vi "ATSh_WaitNextAsyncBufferComplete.vi"(8 "uTimeout_ms":u32, 9 "uBytesPerBuffer":u32, 10 "pBuffer_In":u16[](array[numeric]), 11 "Handle":u32) -> (0 "Return Code":u32, 2 "pBuffer_Out":u16[](array[numeric]), 3 "Handle_Out":u32)   [LabVIEW 2015]
doc: "_____AlazarTech, Scope_____\n\nWait for an asynchronous transfer from on-board to host memory to complete."
uses:
  ATSApi.dll
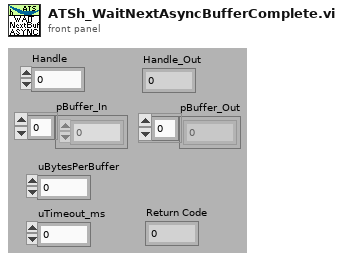
[diagram p1: front panel]
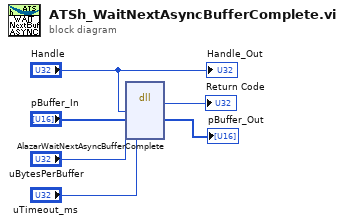
[diagram p0: block diagram]
diagram:
  n1 = dll-call lib="C:/IntensityOCT/trunk/ATSApi.dll" fn="AlazarWaitNextAsyncBufferComplete"("Handle"="Handle", "pBuffer"="pBuffer_In", "uBytesPerBuffer"="uBytesPerBuffer", "uTimeout_ms"="uTimeout_ms") -> (→"Return Code":u32, "pBuffer"=→"pBuffer_Out":u16[])  [unwired: 6 in, 2 out]
  "Handle_Out" <- "Handle"
